vi "Watflow F4 Analog Input.vi"() -> ()   [LabVIEW 2010]
doc: "This VI sets the analog input sensor and other options.\n\nNote: It represents the <B>Main>Setup>Analog Input x</B> menu of the controller."
uses:
  SubVIs/Watflow F4/Watflow F4.lvlib
panel:
  in  "Units (0: Temperature)":u16(ring) items=["Temperature", "% rh", "Psi", "Units"]
  in  "Altitude (0: 0 to 2499 ft)":i16(ring) items=["0 to 2499 ft", "2500 to 4999 ft", "5000 ft and above"]
  in  "Scale High (1500.0)":dbl=1500.0 format="%.2f"
  in  "Scale Low (32.0)":dbl=32.0 format="%.2f"
  in  "Error Latch (0: Self Clear)":u16(ring) items=["Self Clear", "Latch"]
  in  "Filter Time (0.0)":dbl format="%.2f"
  in  "Calibration Offset (0.0)":dbl format="%.2f"
  in  "Set Point High Limit (1500.0)":dbl=1500.0 format="%.2f"
  in  "Set Point Low Limit (32.0)":dbl=32.0 format="%.2f"
  in  "Decimal Point (0: 0)":u16(ring) items=["0", "0.0", "0.00 process", "0.000 process"]
  in  "Type (0: J)":u16(ring) items=["J", "K", "T", "E", "N", "C", "D", "PT2", "R", "S", "B", "100 ohm DIN", "100 ohm JIS", "4 to 20 mA", "0 to 20 mA", "0 to 5 V", "1 to 5 V", "0 to 10 V", "0 to 50 mV", "Vaisala 0 to 5 V", "Vaisala 0 to 10 V", "Vaisala 0 to 20 mA", "Rotronics 0 to 5 V", "500 ohm DIN", "500 ohm JIS", "1000 ohm DIN", "1000 ohm JIS"]
  in  "Sensor (0: Thermocouple)":u16(ring) items=["Thermocouple", "RTD", "Process", "Wet Bulb - Dry Bulb", "Off"]
  in  "Analog Input (1)":i16=1
  in  "Unit Address (1)":u8=1
  in  "Instrument Resource Name":refnum<visa-resource-name>
  in  "error in (no error)":errorcluster
  # "© 2005 National Instruments.  ALL RIGHTS RESERVED."
  # "WATLOW F4 Series"
  # "Main > Setup > Analog Input x"
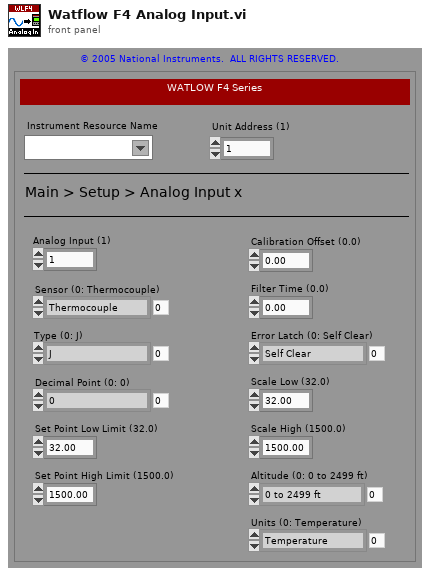
[diagram p1: front panel]
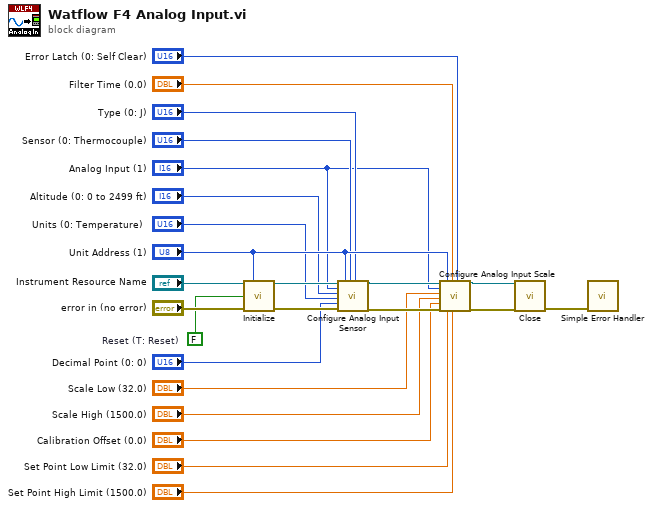
[diagram p0: block diagram]
diagram:
  w21 = FALSE  # Reset (T: Reset)
  n1 = call "Initialize.vi"("VISA resource name"="Instrument Resource Name", "Unit Address (1)"="Unit Address (1)", "Reset (T: Reset)"=w21, "error in (no error)"="error in (no error)") -> ("VISA resource name out"=w15:refnum<visa-resource-name>, "error out"=w20:errorcluster)  [unwired: 10 in]
  n2 = call "Configure Analog Input Sensor.vi"("VISA resource name"=w15, "Analog Input (1)"="Analog Input (1)", "Altitude (0: 0 to 2499 ft)"="Altitude (0: 0 to 2499 ft)", "Units (0: Temperature)"="Units (0: Temperature)", "Decimal Point (0: 0)"="Decimal Point (0: 0)", "error in (no error)"=w20, "Unit Address (1)"="Unit Address (1)", "Sensor (0: Thermocouple)"="Sensor (0: Thermocouple)", "Type (0: J)"="Type (0: J)") -> ("VISA resource name out"=w16:refnum<visa-resource-name>, "error out"=w19:errorcluster)  [unwired: 9 in]
  n3 = call "Configure Analog Input Scale.vi"("VISA resource name"=w16, "Analog Input (1)"="Analog Input (1)", "Scale Low (32.0)"="Scale Low (32.0)", "Scale High (1500.0)"="Scale High (1500.0)", "Calibration Offset (0.0)"="Calibration Offset (0.0)", "error in (no error)"=w19, "Unit Address (1)"="Unit Address (1)", "Set Point Low Limit (32.0)"="Set Point Low Limit (32.0)", "Filter Time (0.0)"="Filter Time (0.0)", "Set Point High Limit (1500.0)"="Set Point High Limit (1500.0)", "Error Latch (0: Self Clear)"="Error Latch (0: Self Clear)") -> ("VISA resource name out"=w17:refnum<visa-resource-name>, "error out"=w18:errorcluster)  [unwired: 7 in]
  n4 = call "Close.vi"("VISA resource name"=w17, "error in (no error)"=w18) -> ("error out"=w22:errorcluster)  [unwired: 13 in]
  n5 = call <vilib>:"Simple Error Handler.vi"("error in (no error)"=w22) -> ()  [unwired: 4 in, 5 out]
